vi "ACQUIS_FREQ.vi"(1 "sample mode":i32(ring)=10178 items=["Finite Samples"=10178, "Continuous Samples"=10123, "Hardware Timed Single Point"=12522], 4 "physical channels":tag="Dev1/ai0") -> (2 "Campioni al secondo":dbl=10000.0 min=0.0 max=250000.0 format="%#.4f")   [LabVIEW 2014]
doc: "Acquisisce un canale emntre genera un sinusoide\n(per le 6221 occorre cambiare il vettore Fondo scala)\n\nFM & ADL 2007, vers. 10/2012\nvers. 10/2013 per versione 8.6"
uses:
  <vilib>/DAQmx/write.llb/DAQmx Write (Analog 1D DBL 1Chan NSamp).vi
  <vilib>/DAQmx/read.llb/DAQmx Read (Analog Wfm 1Chan NSamp).vi
  <vilib>/DAQmx/create/channels.llb/DAQmx Create Channel (AO-Voltage-Basic).vi
  <vilib>/DAQmx/create/channels.llb/DAQmx Create Channel (AI-Voltage-Basic).vi
  <vilib>/DAQmx/configure/timing.llb/DAQmx Timing (Sample Clock).vi
  <vilib>/DAQmx/miscellaneous.llb/DAQmx Fill In Error Info.vi
  <vilib>/Waveform/WDTFileIO.llb/Export Waveform To Spreadsheet File.vi
  <vilib>/measure/NI_MABase.lvlib
  <resource>/objmgr/daqmx.rc
panel:
  out "UGBW":dbl format="%.2e"
  out "Valor medio":dbl format="%#.3g"
  in  "Guadagno del \npartitore":dbl=1000.0 format="%_3e"
  out "Guadagno":dbl format="%#.0f"
  in  "esci":bool
  in  "N. periodi":dbl(ring)=5.0 items=["2"=2.0, "5"=5.0, "10"=10.0, "20"=20.0, "30"=30.0]
  in  "Frequenza (Hz)":dbl=500.0 min=0.1 max=10000.0 step=100.0
  in  "Offset (V)":dbl=0.2 min=-10.0 max=10.0 step=0.01
  in  "Ampiezza (V)":dbl=0.02 min=0.01 max=10.0 step=0.05
  in  "FScala":dbl(ring)=10.0 items=["10"=10.0, "5"=5.0, "0.5"=0.5, "0.05"=0.05]
  in  "SALVA I DATI SU FILE":bool=TRUE caption="ON\nOFF"
  out "V(t)":waveform(dbl)(graph)
  out "Intervallo usato":dbl format="%.2e"
  # "NO\nSI"
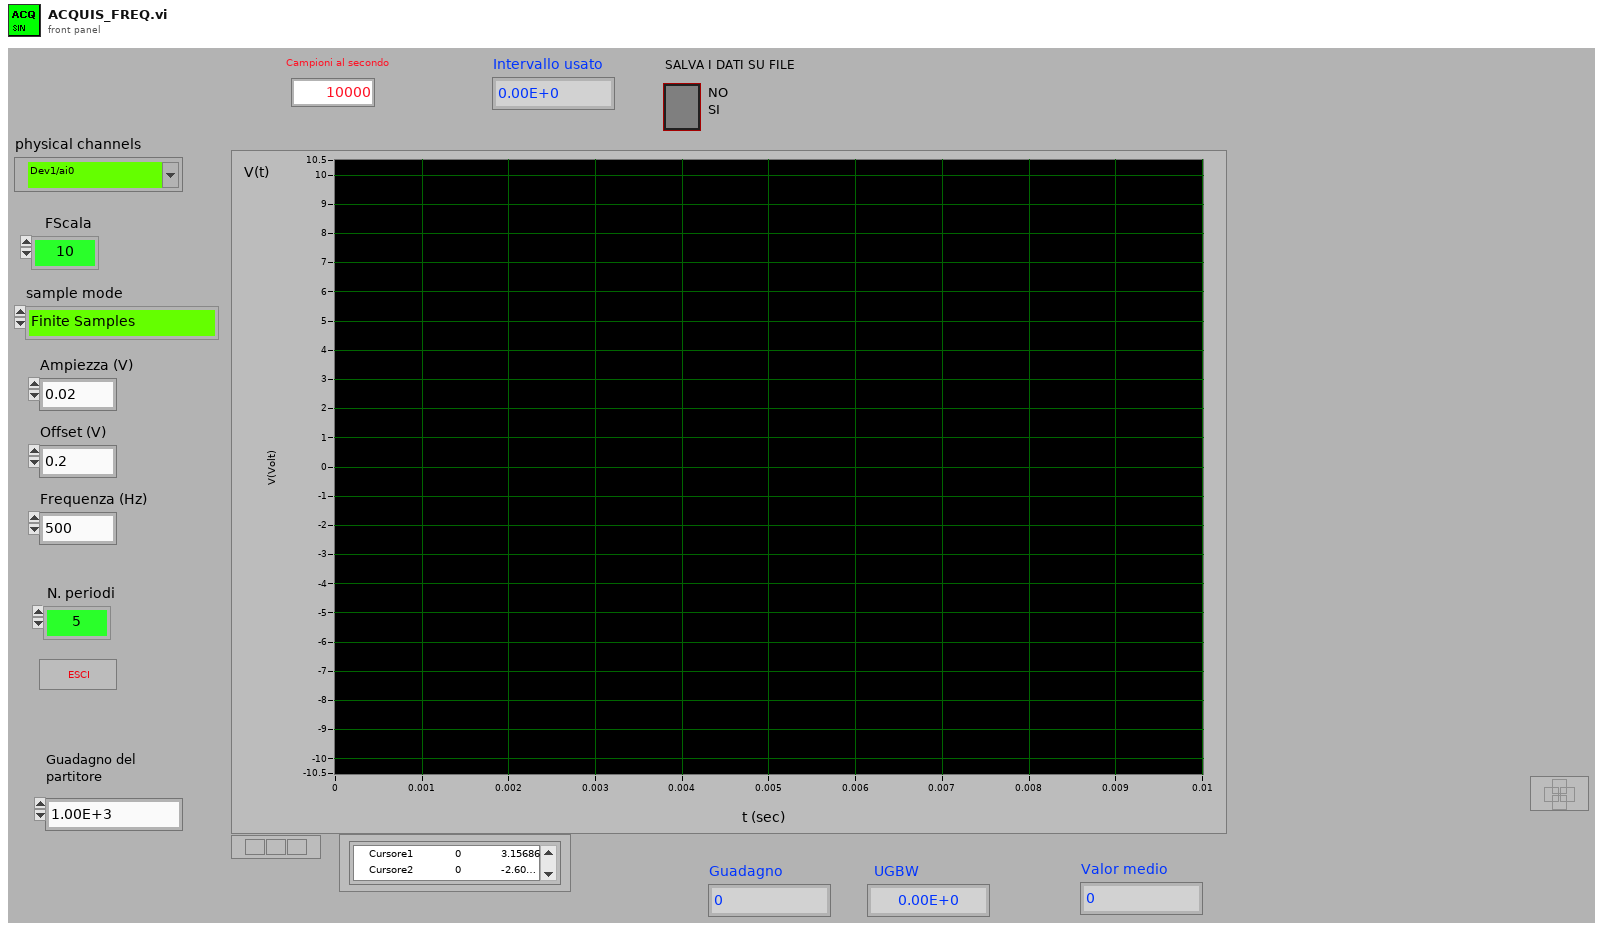
[diagram p1: front panel]
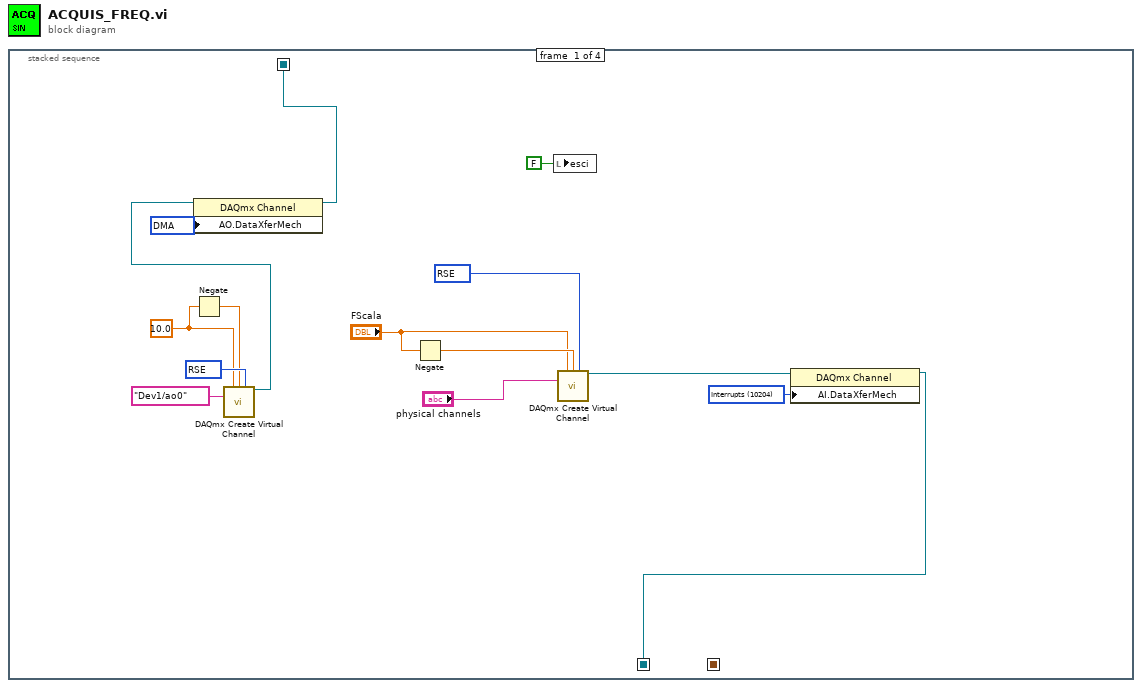
[diagram p0: block diagram]
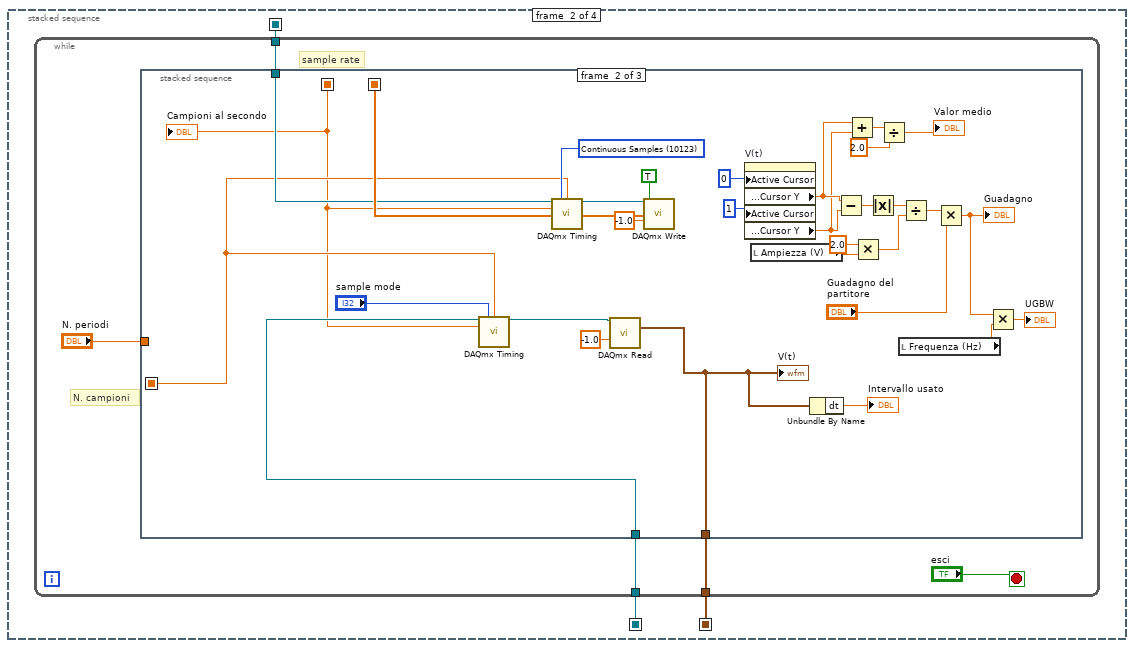
[diagram p2: hidden frame]
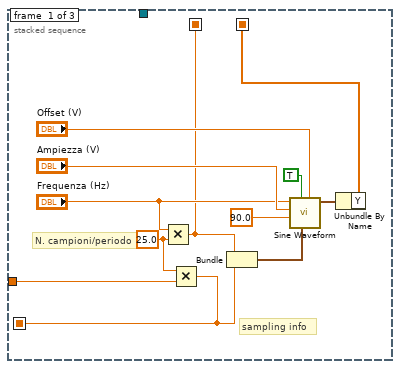
[diagram p3: hidden frame]
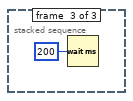
[diagram p4: hidden frame]
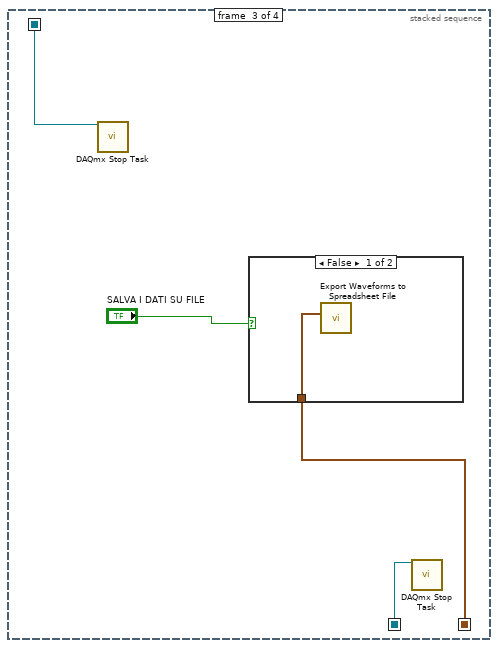
[diagram p5: hidden frame]
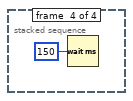
[diagram p7: hidden frame]
diagram:
  n1 = stacked-sequence {
    seq-local: [_ w18 _ _] -> [_ _ w70 _]
    seq-local: [w1 _ _ _] -> [_ w16 w69 _]
    seq-local: [w4 _ _ _] -> [_ w17 w68 _]
    frame #0 {
      w3 = 10054 items=["DMA"=10054, "Interrupts"=10204, "Programmed I/O"=10264, "USB Bulk"=12590] ("AO.DataXferMech")
      w6 = 10204 items=["DMA"=10054, "Interrupts"=10204, "Programmed I/O"=10264, "USB Bulk"=12590] ("AO.DataXferMech")
      w11 = 10083 items=["default"=-1, "RSE"=10083, "NRSE"=10078, "Differential"=10106, "Pseudodifferential"=12529] ("input terminal configuration")
      w13 = 10.0 ("maximum value")
      w14 = 10083 items=["Default"=-1, "RSE"=10083, "Differential"=10106, "Pseudodifferential"=12529] ("output terminal configuration")
      n2 = Negate(x=w13) -> (-x=w12:dbl)
      n3 = call-poly <vilib>:"DAQmx Create Virtual Channel.vi"("maximum value"=w13, "minimum value"=w12, "output terminal configuration"=w14, "physical channels"=tag "Dev1/ao0") -> ("task out"=w2:refnum<k21>)  [unwired: 5 in, 6 out]
      n4 = property class="DAQmx Channel"(reference=w2, "AO.DataXferMech"=w3) -> (reference out=w1:refnum<k21>)  [unwired: 1 in, 1 out]
      n5 = Negate(x="FScala") -> (-x=w9:dbl)
      n6 = local write "esci"(FALSE ("esci")) -> ()
      n7 = call-poly <vilib>:"DAQmx Create Virtual Channel.vi"("maximum value"="FScala", "minimum value"=w9, "input terminal configuration"=w11, "physical channels"="physical channels") -> ("task out"=w5:refnum<k21>)  [unwired: 5 in, 6 out]
      n8 = property class="DAQmx Channel"(reference=w5, "AI.DataXferMech"=w6) -> (reference out=w4:refnum<k21>)  [unwired: 1 in, 1 out]
    }
    frame #1 {
      n9 = while {
        tunnel: [w23] -> w18
        tunnel: w17 -> [w22]
        tunnel: w16 -> [w21]
        stop <- "esci" stop-if-true
        # "N. campioni"
        # "sample rate"
        n10 = stacked-sequence {
          seq-local: [w30 _ _] -> [_ w57 _]
          seq-local: [w28 _ _] -> [_ w54 _]
          seq-local: [w26 _ _] -> [_ w55 _]
          tunnel: [_ w62 _] -> w23
          tunnel: w22 -> [_ w61 _]
          tunnel: w21 -> [_ w56 _]
          tunnel: "N. periodi" -> [w24 _ _]
          frame #0 {
            w25 = 25.0
            # "N. campioni/periodo"
            # "sampling info"
            n11 = Multiply(x="Frequenza (Hz)", y=w25) -> (x*y=w28:dbl)
            n12 = Multiply(x=w25, y=w24) -> (x*y=w26:dbl)
            n13 = Bundle(w28, w26) -> (w27:cluster{dbl, dbl})  [unwired: 1 out]
            n14 = call <vilib>:"Sine Waveform.vi"("offset"="Offset (V)", "sampling info"=w27, "reset signal"=TRUE, "phase"=90.0, "amplitude"="Ampiezza (V)", "frequency"="Frequenza (Hz)") -> ("signal out"=w35:waveform(dbl))  [unwired: 1 in, 4 out]
            n15 = Unbundle By Name(w35) -> ("Y"=w30:dbl[])
          }
          frame #1 {
            w58 = 10123 items=["Finite Samples"=10178, "Continuous Samples"=10123, "Hardware Timed Single Point"=12522] ("sample mode")
            n16 = call-poly <vilib>:"DAQmx Timing.vi"("task/channels in"=w61, "sample mode"="sample mode", "samples per channel"=w55, "rate"=w54) -> ("task out"=w65:refnum<k21>)  [unwired: 3 in, 8 out]
            n17 = call-poly <vilib>:"DAQmx Timing.vi"("task/channels in"=w56, "sample mode"=w58, "samples per channel"=w55, "rate"=w54) -> ("task out"=w59:refnum<k21>)  [unwired: 3 in, 8 out]
            n18 = call-poly <vilib>:"DAQmx Read.vi"("task/channels in"=w65, "timeout"=-1.0) -> ("data"=w62:waveform(dbl))  [unwired: 2 in, 11 out]
            "V(t)" <- w62
            n19 = call-poly <vilib>:"DAQmx Write.vi"("task/channels in"=w59, "auto start"=TRUE, "data"=w57, "timeout"=-1.0) -> ()  [unwired: 1 in, 11 out]
            n20 = property on="V(t)" class="WFGraph (strict)"("Active Cursor"=0 ("Cursor.Cursor Index"), "Active Cursor"=1 ("Cursor.Cursor Index")) -> ("Cursor.Cursor Position:Cursor Y"=w43:dbl, "Cursor.Cursor Position:Cursor Y"=w42:dbl)  [unwired: 2 in, 2 out]
            n21 = local read "Ampiezza (V)"() -> (w49:dbl)
            n22 = Unbundle By Name(w62) -> ("dt"=→"Intervallo usato":dbl)
            n23 = Subtract(x=w43, y=w42) -> (x-y=w51:dbl)
            n24 = Add(x=w43, y=w42) -> (x+y=w41:dbl)
            n25 = Multiply(x=2.0, y=w49) -> (x*y=w47:dbl)
            n26 = Absolute Value(x=w51) -> (abs(x)=w50:dbl)
            n27 = Divide(x=w41, y=2.0) -> (x/y=→"Valor medio":dbl)
            n28 = local read "Frequenza (Hz)"() -> (w36:dbl)
            n29 = Divide(x=w50, y=w47) -> (x/y=w48:dbl)
            n30 = Multiply(x=w48, y="Guadagno del \npartitore") -> (x*y=w37:dbl)
            "Guadagno" <- w37
            n31 = Multiply(x=w37, y=w36) -> (x*y=→"UGBW":dbl)
            "Campioni al secondo" <- w54
          }
          frame #2 {
            n32 = Wait (ms)(milliseconds to wait=u32 200) -> ()  [unwired: 1 out]
          }
        }
      }
    }
    frame #2 {
      n33 = call <vilib>:"DAQmx Stop Task.vi"("task/channels in"=w69) -> ()  [unwired: 1 in, 14 out]
      n34 = case shown="False" "SALVA I DATI SU FILE" {
        tunnel: w70 -> [w72 _]
        frame False {
          n35 = call-poly <vilib>:"Export Waveforms to Spreadsheet File.vi"("waveform"=w72) -> ()  [unwired: 6 in, 5 out]
        }
        frame True {
        }
      }
      n36 = call <vilib>:"DAQmx Stop Task.vi"("task/channels in"=w68) -> ()  [unwired: 1 in, 14 out]
    }
    frame #3 {
      n37 = Wait (ms)(milliseconds to wait=u32 150) -> ()  [unwired: 1 out]
    }
  }
